vi "CLD 4 Event Structure Timer Front Panel.vi"() -> ()   [LabVIEW 2019]
doc: "CLD 4 Challenge Exercise"
panel:
  out "Error Out":errorcluster
  in  "Error In":errorcluster
  out "Bit 4":bool
  out "Bit 3":bool
  out "Bit 2":bool
  out "Bit 1":bool
  out "Time Has Elapsed":bool
  out "Elapsed Time":string
  in  "Auto Reset":bool=TRUE
  in  "Reset Button":bool
  in  "Stop VI":bool
  in  "Time Target (s)":dbl=4.0
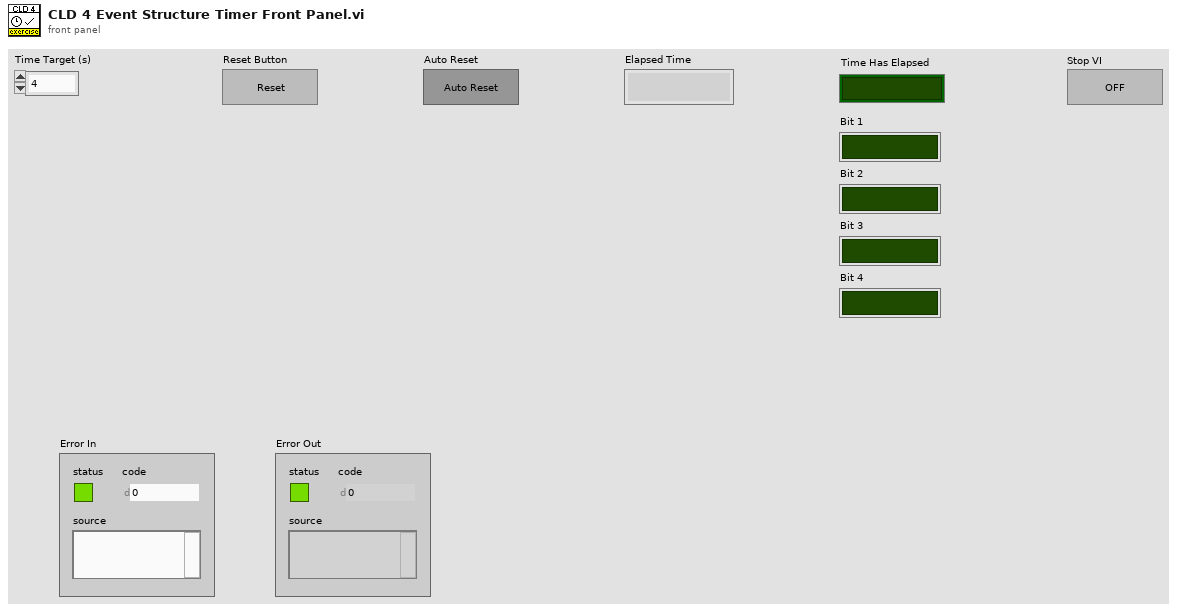
[diagram p1: front panel]
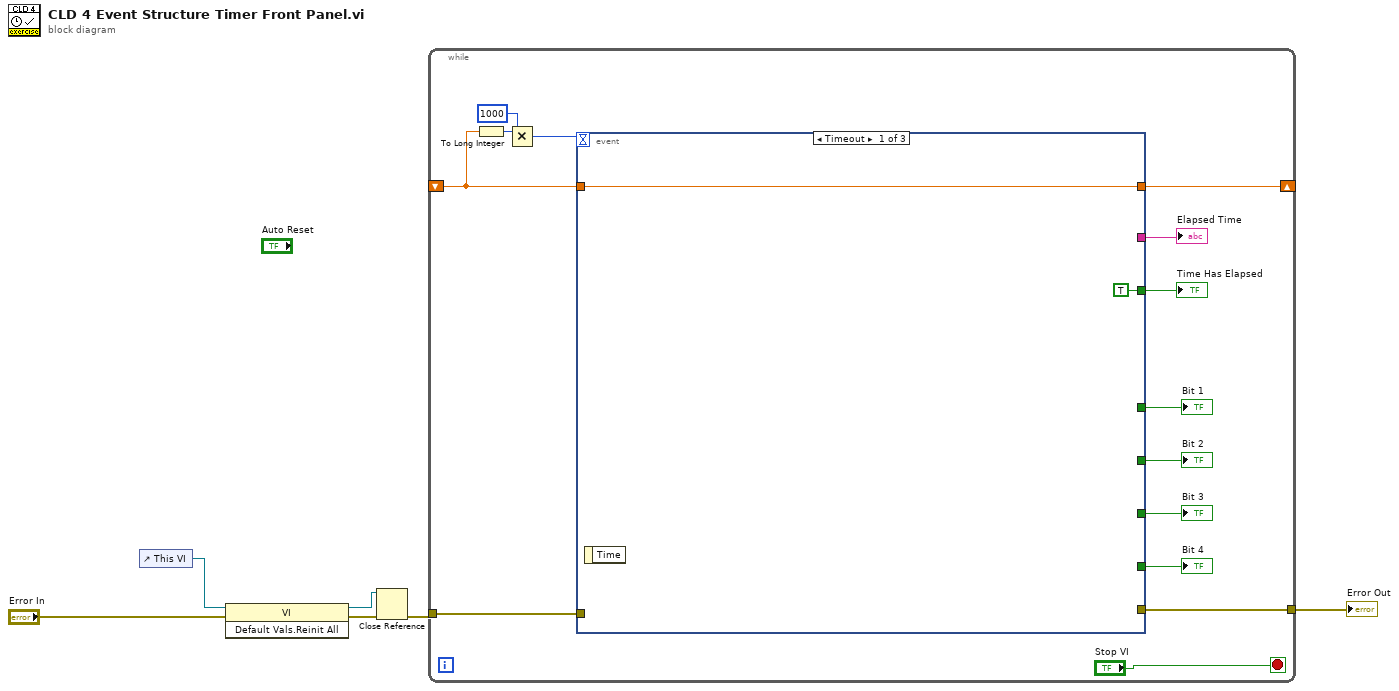
[diagram p0: block diagram]
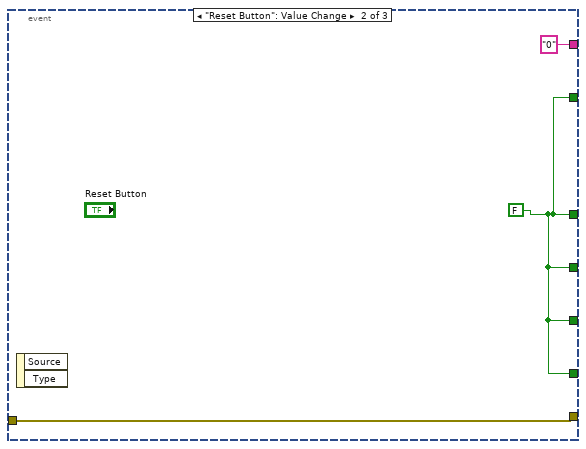
[diagram p2: hidden frame]
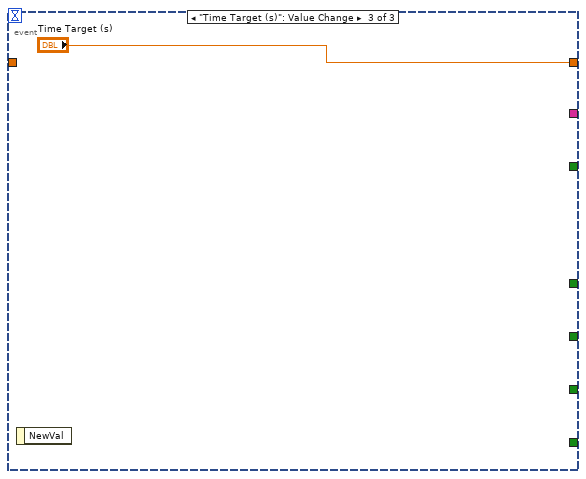
[diagram p3: hidden frame]
diagram:
  n1 = control-ref of="This VI"() -> (w4:refnum<vi>)
  n2 = invoke class="VI" method="Default Vals.Reinit All"(reference=w4, error in="Error In") -> (reference out=w3:refnum<vi>, error out=w5:errorcluster)  [unwired: 1 in, 1 out]
  n3 = Close Reference(reference=w3, error in (no error)=w5) -> (error out=w2:errorcluster)
  n4 = while {
    shift-right: [w17] -> _
    shift-left: _ -> [w16]
    tunnel: w2 -> [w14]
    tunnel: [w13] -> w6
    stop <- "Stop VI" stop-if-true
    n5 = To Long Integer(number=w16) -> (32bit integer=w20:i32)
    n6 = Multiply(x=w20, y=1000) -> (x*y=w18:i32)
    n7 = event shown="[0] Timeout" {
      selector: _ -> [_ _ _]
      dyn-events: _ -> [_ _ _]
      timeout: w18 -> [_ _ _]
      tunnel: [w22 _ "Time Target (s)"] -> w17
      tunnel: w16 -> [w22 _ _]
      tunnel: [_ w25 _] -> w13
      tunnel: w14 -> [_ w25 _]
      tunnel: [_ w24 _] -> w12
      tunnel: [_ w24 _] -> w11
      tunnel: [_ w24 _] -> w10
      tunnel: [_ w24 _] -> w9
      tunnel: [TRUE ("Bit 1") w24 _] -> w8
      tunnel: [_ "0" ("Elapsed Time") _] -> w7
      event Timeout {
        n8 = event-data() -> ()  [unwired: 1 in, 1 out]
      }
      event "Reset Button": Value Change {
        w24 = FALSE ("Bit 1")
        n9 = event-data() -> ()  [unwired: 1 in, 2 out]
      }
      event "Time Target (s)": Value Change {
        n10 = event-data() -> ()  [unwired: 1 in, 1 out]
      }
    }
    "Bit 1" <- w12
    "Bit 2" <- w11
    "Bit 3" <- w10
    "Bit 4" <- w9
    "Time Has Elapsed" <- w8
    "Elapsed Time" <- w7
  }
  "Error Out" <- w6
